vi "z_N[Lambda_tau,T,W,t_0]_Analytical.vi"(4 "Use z[0]":bool, 6 "t0":ext, 7 "Harmonic f":ext, 8 "N":i32, 9 "W":ext, 10 "T":ext, 11 "tau":ext) -> (3 "z_n,N,W(tau)":cxt)   [LabVIEW 2021, in "Phasor.lvlib"]
uses:
  Phasor.lvlib
  d7224bb0-7287-4d58-abbb-d1bd0f91def9.vi
  9cc972f5-8a98-42e2-8998-2ddda7d4f1f6.vi
  d7224bb0-7287-4d58-abbb-d1bd0f91def9.vi/8a80743f-1319-44c8-96b0-3ef8fc688731.vi
  d7224bb0-7287-4d58-abbb-d1bd0f91def9.vi/931f4f8f-d8c6-4056-833f-5c8fe97b24b9.vi
  9cc972f5-8a98-42e2-8998-2ddda7d4f1f6.vi/8a80743f-1319-44c8-96b0-3ef8fc688731.vi
  9cc972f5-8a98-42e2-8998-2ddda7d4f1f6.vi/931f4f8f-d8c6-4056-833f-5c8fe97b24b9.vi
  Math/ix/ix (EXT).vi
  Math/Math.lvlib
  22872093-43a4-40af-9bc9-9c64a134b50d.vi
  14c61276-7c1d-4dbf-adfa-5aadda4cd48c.vi
  51be3234-f280-4696-b9d2-a53dd0ed5f61.vi
  cc992cef-98b9-4ce6-98ee-904778ecd6ff.vi
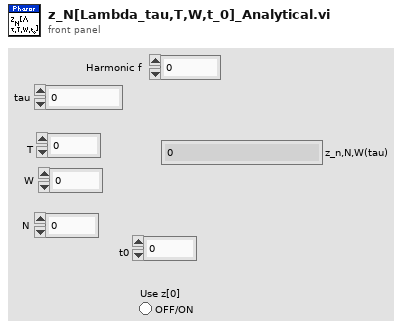
[diagram p1: front panel]
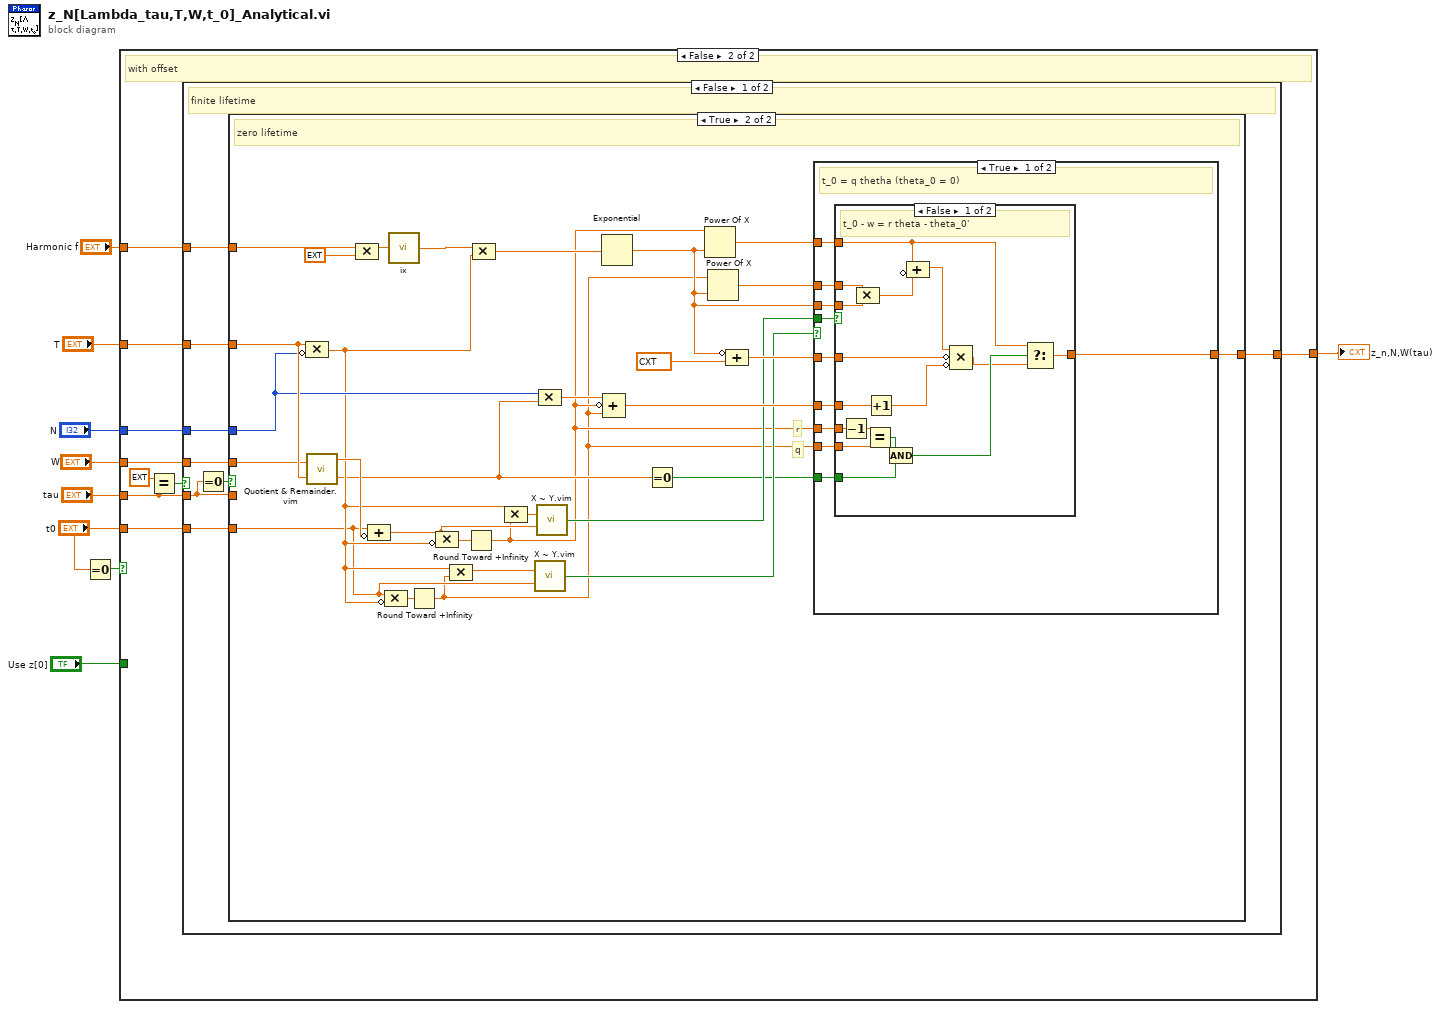
[diagram p0: block diagram]
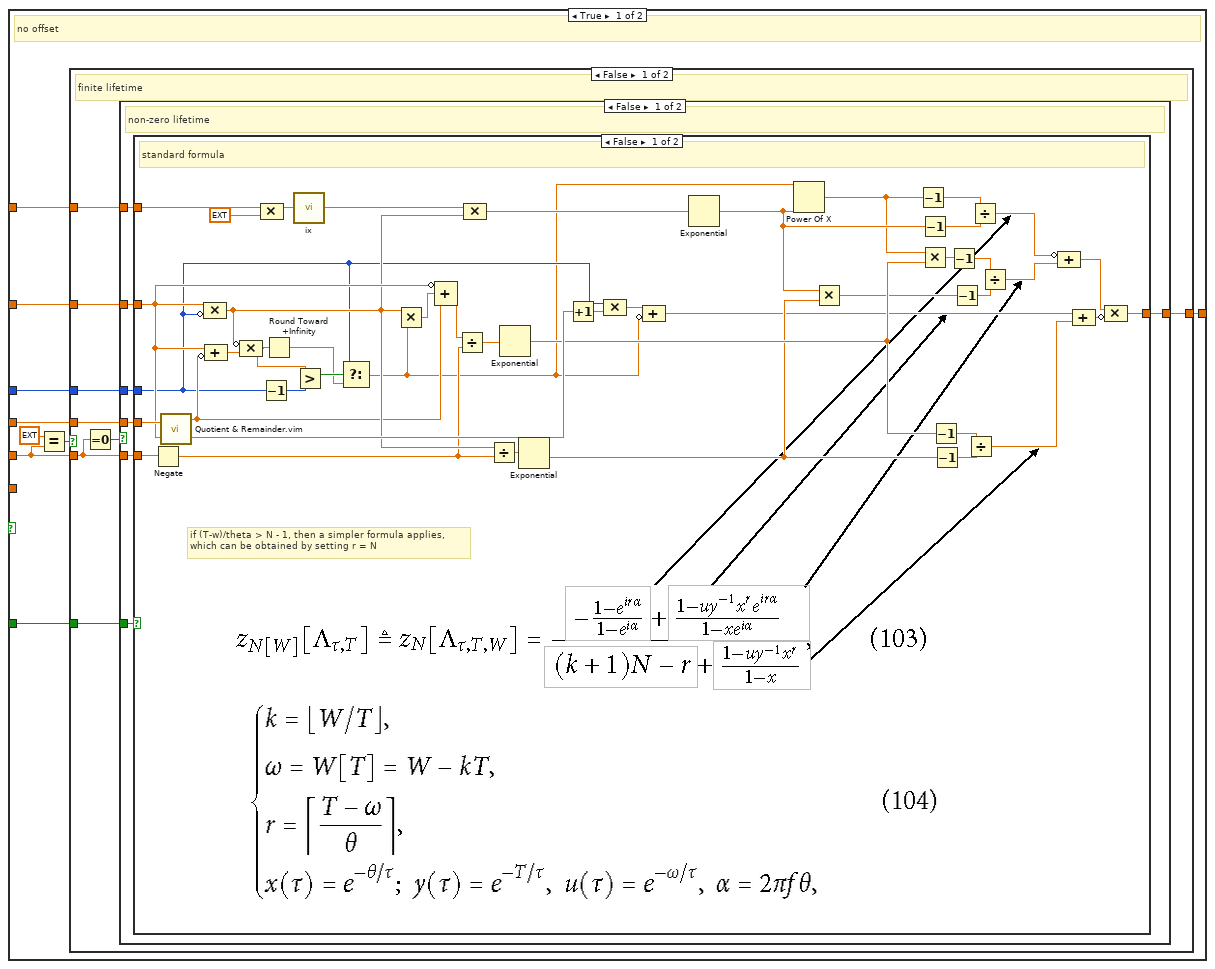
[diagram p2: hidden frame]
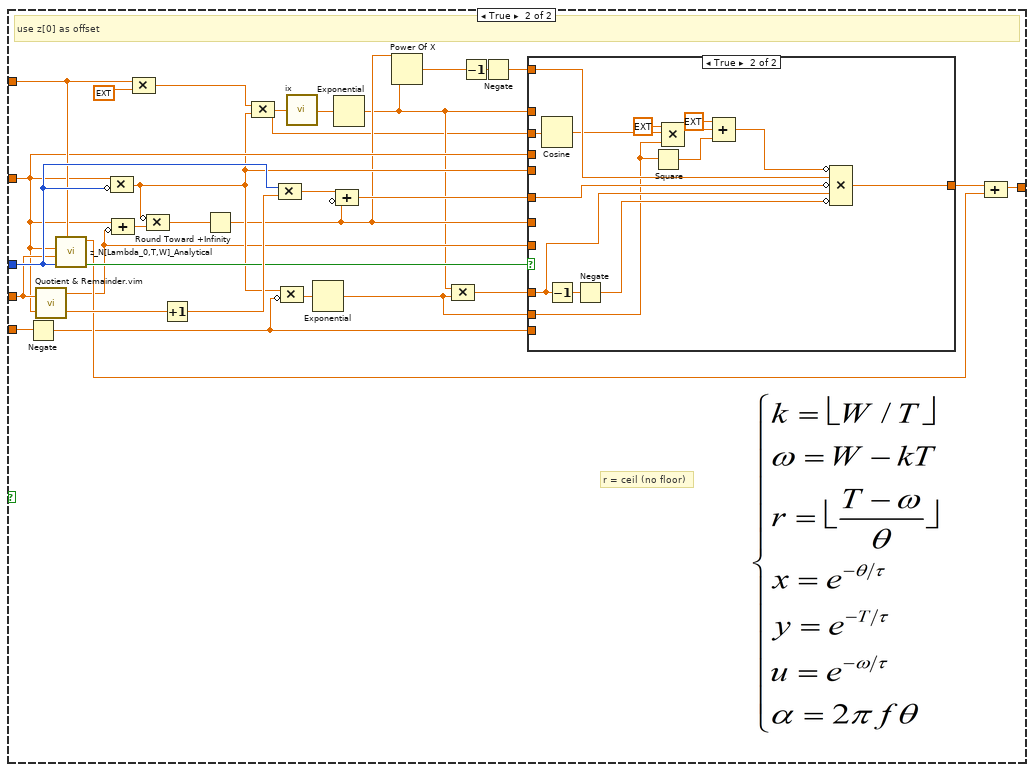
[diagram p3: hidden frame]
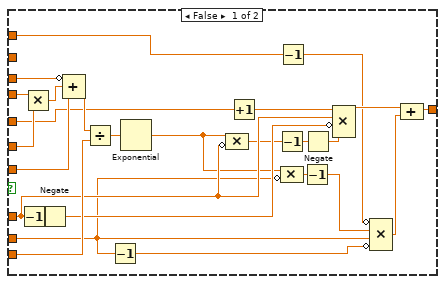
[diagram p4: hidden frame]
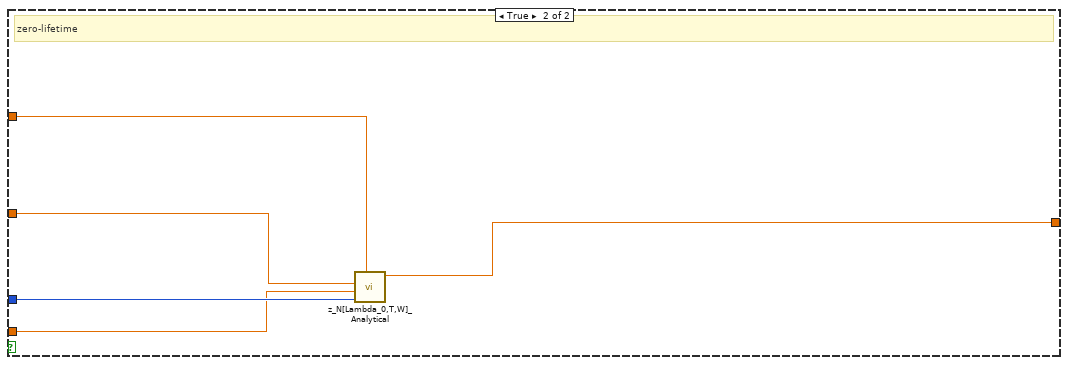
[diagram p5: hidden frame]
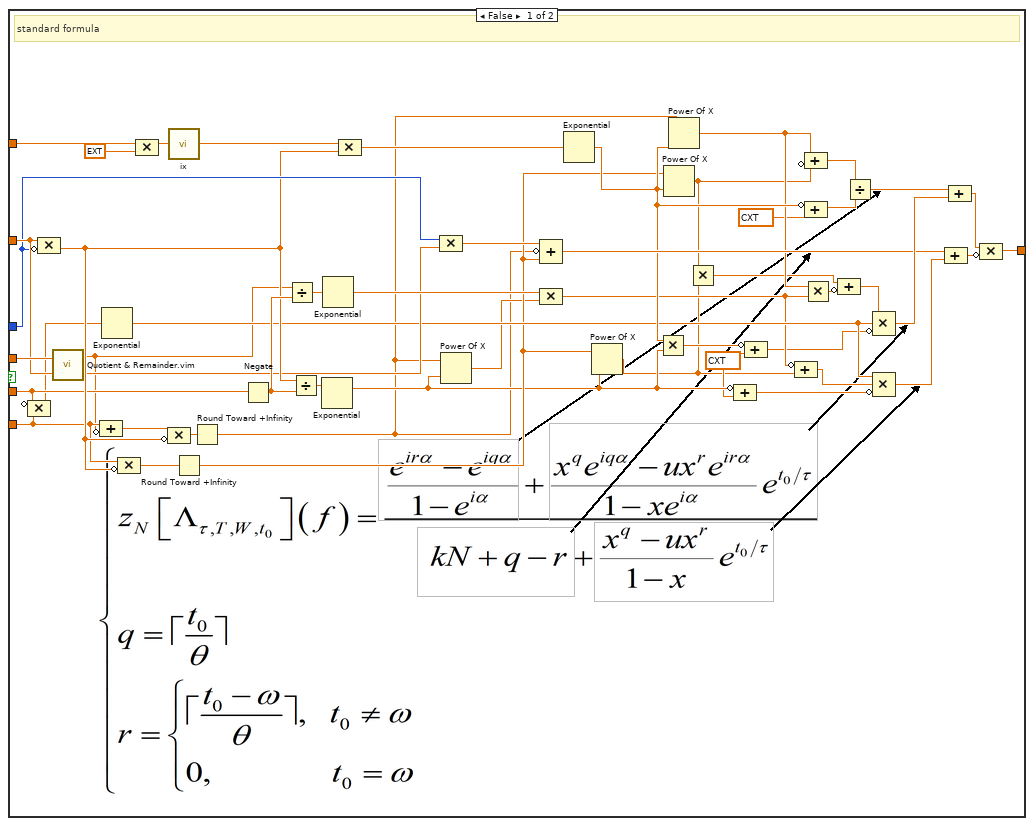
[diagram p7: hidden frame]
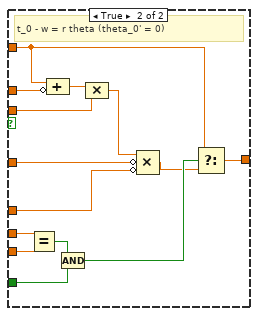
[diagram p8: hidden frame]
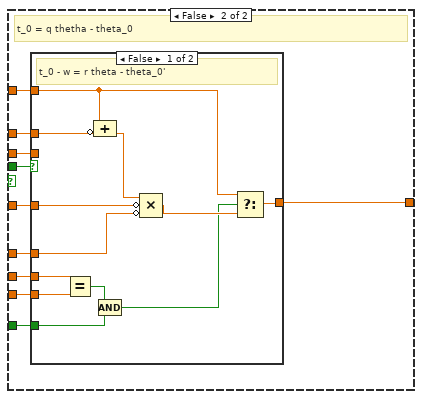
[diagram p9: hidden frame]
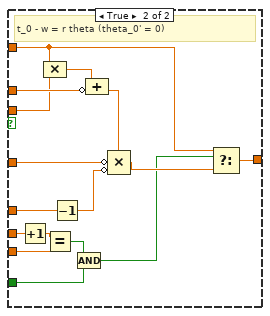
[diagram p10: hidden frame]
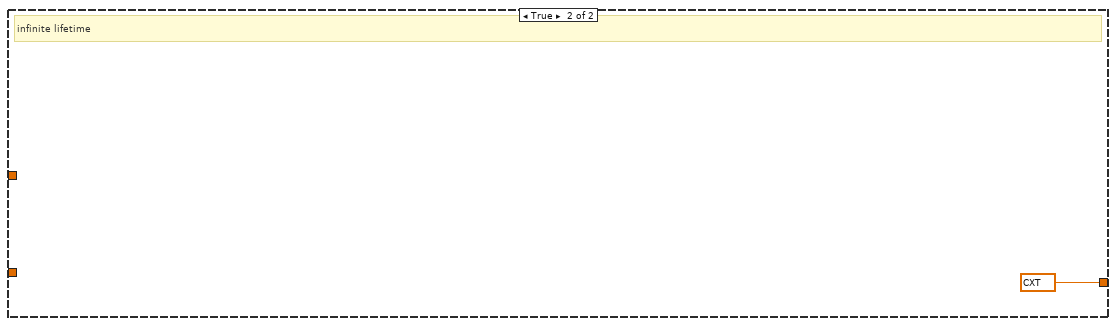
[diagram p11: hidden frame]
diagram:
  n1 = Equal To 0?(x="t0") -> (x = 0?=w2:bool)
  n2 = case shown="False" w2 {
    tunnel: "tau" -> [w13 w159]
    tunnel: "Harmonic f" -> [w18 w157]
    tunnel: [w17 w158] -> w7
    tunnel: "W" -> [w16 w156]
    tunnel: "T" -> [w14 w155]
    tunnel: "N" -> [w15 w154]
    tunnel: "t0" -> [_ w153]
    tunnel: "Use z[0]" -> [w10 _]
    frame True {
      # "no offset"
      n3 = Equal?(x=ext inf, y=w13) -> (x = y?=w11:bool)
      n4 = case shown="False" w11 {
        tunnel: w18 -> [w21 _]
        tunnel: [w26 _] -> w17
        tunnel: w16 -> [w25 _]
        tunnel: w15 -> [w24 _]
        tunnel: w14 -> [w23 _]
        tunnel: w13 -> [w22 _]
        tunnel: w10 -> [w19 _]
        frame False {
          # "finite lifetime"
          n5 = Equal To 0?(x=w22) -> (x = 0?=w20:bool)
          n6 = case shown="False" w20 {
            tunnel: [w33 w151] -> w26
            tunnel: w25 -> [w32 w148]
            tunnel: w24 -> [w31 w152]
            tunnel: w23 -> [w30 w149]
            tunnel: w22 -> [w29 _]
            tunnel: w21 -> [w28 w150]
            tunnel: w19 -> [w27 _]
            frame False {
              # "non-zero lifetime"
              n7 = case shown="False" w27 {
                tunnel: [w77 w93] -> w33
                tunnel: w32 -> [w76 w96]
                tunnel: w31 -> [w49 w98]
                tunnel: w30 -> [w60 w86]
                tunnel: w29 -> [w57 w101]
                tunnel: w28 -> [w46 w97]
                frame False {
                  # "if (T-w)/theta > N - 1, then a simpler formula applies,\nwhich can be obtained by setting r = N"
                  # "standard formula"
                  n8 = Negate(x=w57) -> (-x=w54:ext)
                  n9 = call "Quotient & Remainder.vim"("y"=w60, "x"=w76) -> ("E(x/y)"=w75:ext, "x - E(x/y)y"=w55:ext)
                  n10 = Compound Arithmetic op=MULTIPLY(w60, invert w49) -> (w58:ext)
                  n11 = Compound Arithmetic op=ADD(w60, invert w55) -> (w56:ext)
                  n12 = Compound Arithmetic op=MULTIPLY(invert w58, w56) -> (w47:ext)
                  n13 = Compound Arithmetic op=MULTIPLY(w46, ext 6.283185307179586477) -> (w45:ext)
                  n14 = Decrement(x=w49) -> (x-1=w52:i32)
                  n15 = Round Toward +Infinity(x=w47) -> (ceil(x): smallest int >= x=w50:ext)
                  n16 = call-poly "ix.vi"("x (1)"=w45) -> ("i.(x)"=w44:cxt)
                  n17 = Greater?(x=w47, y=w52) -> (0:w51:bool)
                  n18 = Select(t=w49, s=w51, f=w50) -> (s? t:f=w48:ext)
                  n19 = Multiply(x=w58, y=w48) -> (x*y=w43:ext)
                  n20 = Compound Arithmetic op=ADD(invert w60, w43, w55) -> (w42:ext)
                  n21 = Divide(x=w42, y=w54) -> (x/y=w41:ext)
                  n22 = Compound Arithmetic op=MULTIPLY(w44, w58) -> (w59:cxt)
                  n23 = Divide(x=w58, y=w54) -> (x/y=w40:ext)
                  n24 = Exponential(1:w41) -> (0:w72:ext)
                  n25 = Exponential(1:w40) -> (0:w69:ext)
                  n26 = Increment(x=w75) -> (x+1=w68:ext)
                  n27 = Compound Arithmetic op=MULTIPLY(w49, w68) -> (w67:ext)
                  n28 = Compound Arithmetic op=ADD(w67, invert w48) -> (w66:ext)
                  n29 = Exponential(1:w59) -> (0:w65:cxt)
                  n30 = Power Of X(1:w65, 2:w48) -> (0:w63:cxt)
                  n31 = Multiply(x=w65, y=w69) -> (x*y=w37:cxt)
                  n32 = Decrement(x=w63) -> (x-1=w53:cxt)
                  n33 = Decrement(x=w65) -> (x-1=w64:cxt)
                  n34 = Multiply(x=w63, y=w72) -> (x*y=w36:cxt)
                  n35 = Decrement(x=w72) -> (x-1=w35:ext)
                  n36 = Decrement(x=w69) -> (x-1=w34:ext)
                  n37 = Decrement(x=w36) -> (x-1=w39:cxt)
                  n38 = Decrement(x=w37) -> (x-1=w38:cxt)
                  n39 = Divide(x=w35, y=w34) -> (x/y=w71:ext)
                  n40 = Divide(x=w53, y=w64) -> (x/y=w62:cxt)
                  n41 = Divide(x=w39, y=w38) -> (x/y=w74:cxt)
                  n42 = Compound Arithmetic op=ADD(invert w62, w74) -> (w73:cxt)
                  n43 = Compound Arithmetic op=ADD(w66, w71) -> (w61:ext)
                  n44 = Compound Arithmetic op=MULTIPLY(w73, invert w61) -> (w77:cxt)
                }
                frame True {
                  # "r = ceil (no floor)"
                  # "use z[0] as offset"
                  n45 = Negate(x=w101) -> (-x=w82:ext)
                  n46 = call "Quotient & Remainder.vim"("y"=w86, "x"=w96) -> ("E(x/y)"=w107:ext, "x - E(x/y)y"=w83:ext)
                  n47 = call "z_N[Lambda_0,T,W]_Analytical.vi"("Harmonic f"=w97, "N"=w98, "W"=w96, "T"=w86) -> ("(T-w)/theta integer"=w95:bool, "z_n,N,W(0)"=w94:cxt)  [unwired: 6 in]
                  n48 = Compound Arithmetic op=MULTIPLY(w86, invert w98) -> (w85:ext)
                  n49 = Compound Arithmetic op=ADD(w86, invert w83) -> (w100:ext)
                  n50 = Compound Arithmetic op=MULTIPLY(w97, ext 6.283185307179586477) -> (w102:ext)
                  n51 = Compound Arithmetic op=MULTIPLY(invert w85, w100) -> (w99:ext)
                  n52 = Increment(x=w107) -> (x+1=w105:ext)
                  n53 = Round Toward +Infinity(x=w99) -> (ceil(x): smallest int >= x=w84:ext)
                  n54 = Compound Arithmetic op=MULTIPLY(w102, w85) -> (w79:ext)
                  n55 = Compound Arithmetic op=MULTIPLY(w98, w105) -> (w104:ext)
                  n56 = Compound Arithmetic op=MULTIPLY(w85, invert w82) -> (w89:ext)
                  n57 = call-poly "ix.vi"("x (1)"=w79) -> ("i.(x)"=w78:cxt)
                  n58 = Exponential(1:w89) -> (0:w81:ext)
                  n59 = Exponential(1:w78) -> (0:w80:cxt)
                  n60 = Compound Arithmetic op=ADD(w104, invert w84) -> (w91:ext)
                  n61 = Power Of X(1:w80, 2:w84) -> (0:w103:cxt)
                  n62 = Compound Arithmetic op=MULTIPLY(w80, w81) -> (w88:cxt)
                  n63 = Decrement(x=w103) -> (x-1=w92:cxt)
                  n64 = Negate(x=w92) -> (-x=w90:cxt)
                  n65 = case shown="True" w95 {
                    tunnel: w90 -> [_ w147]
                    tunnel: w91 -> [w125 w146]
                    tunnel: w88 -> [w121 w143]
                    tunnel: [w116 w142] -> w87
                    tunnel: w86 -> [w133 _]
                    tunnel: w85 -> [w132 _]
                    tunnel: w84 -> [w126 _]
                    tunnel: w83 -> [w131 _]
                    tunnel: w82 -> [w130 _]
                    tunnel: w81 -> [w112 w136]
                    tunnel: w80 -> [w113 _]
                    tunnel: w79 -> [_ w141]
                    frame False {
                      n66 = Decrement(x=w121) -> (x-1=w123:cxt)
                      n67 = Multiply(x=w132, y=w126) -> (x*y=w129:ext)
                      n68 = Negate(x=w123) -> (-x=w122:cxt)
                      n69 = Compound Arithmetic op=ADD(invert w133, w129, w131) -> (w128:ext)
                      n70 = Divide(x=w128, y=w130) -> (x/y=w127:ext)
                      n71 = Decrement(x=w112) -> (x-1=w111:ext)
                      n72 = Exponential(1:w127) -> (0:w115:ext)
                      n73 = Compound Arithmetic op=MULTIPLY(w115, invert w121) -> (w119:cxt)
                      n74 = Increment(x=w125) -> (x+1=w124:ext)
                      n75 = Decrement(x=w119) -> (x-1=w120:cxt)
                      n76 = Decrement(x=w113) -> (x-1=w108:cxt)
                      n77 = Compound Arithmetic op=MULTIPLY(w115, invert w112) -> (w114:ext)
                      n78 = Decrement(x=w114) -> (x-1=w109:ext)
                      n79 = Negate(x=w120) -> (-x=w118:cxt)
                      n80 = Compound Arithmetic op=MULTIPLY(w124, w121, invert w122, w118) -> (w117:cxt)
                      n81 = Compound Arithmetic op=MULTIPLY(invert w108, w109, w112, invert w111) -> (w110:cxt)
                      n82 = Compound Arithmetic op=ADD(w117, w110) -> (w116:cxt)
                    }
                    frame True {
                      n83 = Cosine(x=w141) -> (cos(x)=w140:ext)
                      n84 = Decrement(x=w143) -> (x-1=w145:cxt)
                      n85 = Negate(x=w145) -> (-x=w144:cxt)
                      n86 = Square(x=w136) -> (x^2=w135:ext)
                      n87 = Compound Arithmetic op=MULTIPLY(ext -2.0 ("value"), w140, w136) -> (w138:ext)
                      n88 = Compound Arithmetic op=ADD(ext 1.0 ("value"), w138, w135) -> (w134:ext)
                      n89 = Compound Arithmetic op=MULTIPLY(invert w134, w147, invert w146, w143, invert w144) -> (w142:cxt)
                    }
                  }
                  n90 = Compound Arithmetic op=ADD(w87, w94) -> (w93:cxt)
                }
              }
            }
            frame True {
              # "zero-lifetime"
              n91 = call "z_N[Lambda_0,T,W]_Analytical.vi"("Harmonic f"=w150, "N"=w152, "W"=w148, "T"=w149) -> ("z_n,N,W(0)"=w151:cxt)  [unwired: 6 in, 1 out]
            }
          }
        }
        frame True {
          # "infinite lifetime"
        }
      }
    }
    frame False {
      # "with offset"
      n92 = Equal?(x=ext inf, y=w159) -> (x = y?=w160:bool)
      n93 = case shown="False" w160 {
        tunnel: w159 -> [w165 _]
        tunnel: [w163 cxt 0.0+0.0i ("z_n,N,W(0)")] -> w158
        tunnel: w157 -> [w168 _]
        tunnel: w156 -> [w167 _]
        tunnel: w155 -> [w166 _]
        tunnel: w154 -> [w164 _]
        tunnel: w153 -> [w162 _]
        frame False {
          # "finite lifetime"
          n94 = Equal To 0?(x=w165) -> (x = 0?=w169:bool)
          n95 = case shown="True" w169 {
            tunnel: [w219 w221] -> w163
            tunnel: w167 -> [w218 w220]
            tunnel: w164 -> [w204 w245]
            tunnel: w166 -> [w207 w247]
            tunnel: w165 -> [w188 _]
            tunnel: w168 -> [w203 w244]
            tunnel: w162 -> [w187 w232]
            frame False {
              w176 = cxt 1.0+0.0i ("value")
              # "standard formula"
              n96 = Compound Arithmetic op=MULTIPLY(invert w188, w187) -> (w186:ext)
              n97 = Compound Arithmetic op=MULTIPLY(w207, invert w204) -> (w196:ext)
              n98 = call "Quotient & Remainder.vim"("y"=w207, "x"=w218) -> ("E(x/y)"=w189:ext, "x - E(x/y)y"=w182:ext)
              n99 = Compound Arithmetic op=ADD(w187, invert w182) -> (w194:ext)
              n100 = Exponential(1:w186) -> (0:w184:ext)
              n101 = Compound Arithmetic op=MULTIPLY(w187, invert w196) -> (w197:ext)
              n102 = Compound Arithmetic op=MULTIPLY(w203, ext 6.283185307179586477) -> (w202:ext)
              n103 = Compound Arithmetic op=MULTIPLY(w194, invert w196) -> (w195:ext)
              n104 = call-poly "ix.vi"("x (1)"=w202) -> ("i.(x)"=w201:cxt)
              n105 = Round Toward +Infinity(x=w197) -> (ceil(x): smallest int >= x=w183:ext)
              n106 = Round Toward +Infinity(x=w195) -> (ceil(x): smallest int >= x=w170:ext)
              n107 = Negate(x=w188) -> (-x=w205:ext)
              n108 = Divide(x=w182, y=w205) -> (x/y=w200:ext)
              n109 = Divide(x=w196, y=w205) -> (x/y=w199:ext)
              n110 = Exponential(1:w199) -> (0:w181:ext)
              n111 = Exponential(1:w200) -> (0:w215:ext)
              n112 = Compound Arithmetic op=MULTIPLY(w201, w196) -> (w206:cxt)
              n113 = Compound Arithmetic op=MULTIPLY(w204, w189) -> (w212:ext)
              n114 = Power Of X(1:w181, 2:w170) -> (0:w179:ext)
              n115 = Compound Arithmetic op=ADD(w212, invert w170, w183) -> (w211:ext)
              n116 = Compound Arithmetic op=MULTIPLY(w215, w179) -> (w180:ext)
              n117 = Exponential(1:w206) -> (0:w193:cxt)
              n118 = Power Of X(1:w181, 2:w183) -> (0:w174:ext)
              n119 = Multiply(x=w193, y=w181) -> (x*y=w178:cxt)
              n120 = Power Of X(1:w193, 2:w183) -> (0:w175:cxt)
              n121 = Power Of X(1:w193, 2:w170) -> (0:w192:cxt)
              n122 = Multiply(x=w175, y=w174) -> (x*y=w172:cxt)
              n123 = Compound Arithmetic op=unknown(invert w181, w176) -> (w198:cxt)
              n124 = Compound Arithmetic op=ADD(invert w178, w176) -> (w177:cxt)
              n125 = Compound Arithmetic op=ADD(invert w180, w174) -> (w185:ext)
              n126 = Multiply(x=w192, y=w180) -> (x*y=w173:cxt)
              n127 = Compound Arithmetic op=ADD(w192, invert w175) -> (w191:cxt)
              n128 = Compound Arithmetic op=ADD(invert w193, cxt 1.0+0.0i ("value")) -> (w210:cxt)
              n129 = Compound Arithmetic op=ADD(w172, invert w173) -> (w171:cxt)
              n130 = Divide(x=w191, y=w210) -> (x/y=w209:cxt)
              n131 = Compound Arithmetic op=MULTIPLY(w171, w184, invert w177) -> (w217:cxt)
              n132 = Compound Arithmetic op=MULTIPLY(w184, w185, invert w198) -> (w214:cxt)
              n133 = Compound Arithmetic op=ADD(w211, w214) -> (w208:cxt)
              n134 = Compound Arithmetic op=ADD(w209, w217) -> (w216:cxt)
              n135 = Compound Arithmetic op=MULTIPLY(w216, invert w208) -> (w219:cxt)
            }
            frame True {
              # "q"
              # "r"
              # "zero lifetime"
              n136 = Compound Arithmetic op=MULTIPLY(w247, invert w245) -> (w233:ext)
              n137 = call "Quotient & Remainder.vim"("y"=w247, "x"=w220) -> ("E(x/y)"=w225:ext, "x - E(x/y)y"=w238:ext)
              n138 = Compound Arithmetic op=MULTIPLY(w244, ext 6.283185307179586477) -> (w243:ext)
              n139 = Compound Arithmetic op=ADD(w232, invert w238) -> (w234:ext)
              n140 = Compound Arithmetic op=MULTIPLY(w232, invert w233) -> (w241:ext)
              n141 = call-poly "ix.vi"("x (1)"=w243) -> ("i.(x)"=w242:cxt)
              n142 = Round Toward +Infinity(x=w241) -> (ceil(x): smallest int >= x=w222:ext)
              n143 = Compound Arithmetic op=MULTIPLY(w234, invert w233) -> (w240:ext)
              n144 = Compound Arithmetic op=MULTIPLY(w233, w222) -> (w231:ext)
              n145 = Round Toward +Infinity(x=w240) -> (ceil(x): smallest int >= x=w223:ext)
              n146 = Compound Arithmetic op=MULTIPLY(w242, w233) -> (w246:cxt)
              n147 = Compound Arithmetic op=MULTIPLY(w233, w223) -> (w235:ext)
              n148 = call "X ~ Y.vim"("X"=w231, "Y"=w232) -> ("X ~= Y?"=w228:bool)  [unwired: 13 in]
              n149 = call "X ~ Y.vim"("X"=w235, "Y"=w234) -> ("X ~= Y?"=w227:bool)  [unwired: 13 in]
              n150 = Compound Arithmetic op=MULTIPLY(w245, w225) -> (w248:ext)
              n151 = Exponential(1:w246) -> (0:w226:cxt)
              n152 = Compound Arithmetic op=ADD(w248, invert w223, w222) -> (w236:ext)
              n153 = Equal To 0?(x=w225) -> (x = 0?=w224:bool)
              n154 = Power Of X(1:w226, 2:w223) -> (0:w239:cxt)
              n155 = Power Of X(1:w226, 2:w222) -> (0:w237:cxt)
              n156 = Compound Arithmetic op=ADD(invert w226, cxt 1.0+0.0i ("value")) -> (w229:cxt)
              n157 = case shown="True" w228 {
                tunnel: w239 -> [w259 w299]
                tunnel: w237 -> [w258 w298]
                tunnel: w227 -> [w257 w297]
                tunnel: w226 -> [w256 w296]
                tunnel: w236 -> [w254 w291]
                tunnel: w229 -> [w255 w292]
                tunnel: w224 -> [w251 w295]
                tunnel: w223 -> [w253 w294]
                tunnel: w222 -> [w252 w293]
                tunnel: [w250 w290] -> w221
                frame True {
                  # "t_0 = q thetha (theta_0 = 0)"
                  n158 = case shown="False" w257 {
                    tunnel: w259 -> [w261 w276]
                    tunnel: w258 -> [w275 w289]
                    tunnel: w256 -> [w274 w287]
                    tunnel: w255 -> [w271 w281]
                    tunnel: w254 -> [w270 w280]
                    tunnel: w253 -> [w266 w286]
                    tunnel: w252 -> [w265 w285]
                    tunnel: w251 -> [w264 w283]
                    tunnel: [w268 w278] -> w250
                    frame False {
                      # "t_0 - w = r theta - theta_0'"
                      n159 = Decrement(x=w266) -> (x-1=w260:ext)
                      n160 = Compound Arithmetic op=MULTIPLY(w275, w274) -> (w273:cxt)
                      n161 = Equal?(x=w260, y=w265) -> (x = y?=w267:bool)
                      n162 = Increment(x=w270) -> (x+1=w269:ext)
                      n163 = Compound Arithmetic op=AND(w267, w264) -> (w263:bool)
                      n164 = Compound Arithmetic op=ADD(w261, invert w273) -> (w272:cxt)
                      n165 = Compound Arithmetic op=MULTIPLY(w272, invert w271, invert w269) -> (w262:cxt)
                      n166 = Select(t=w261, s=w263, f=w262) -> (s? t:f=w268:cxt)
                    }
                    frame True {
                      # "t_0 - w = r theta (theta_0' = 0)"
                      n167 = Equal?(x=w286, y=w285) -> (x = y?=w284:bool)
                      n168 = Compound Arithmetic op=ADD(w276, invert w289) -> (w288:cxt)
                      n169 = Compound Arithmetic op=AND(w284, w283) -> (w279:bool)
                      n170 = Compound Arithmetic op=MULTIPLY(w288, w287) -> (w282:cxt)
                      n171 = Compound Arithmetic op=MULTIPLY(w282, invert w281, invert w280) -> (w277:cxt)
                      n172 = Select(t=w276, s=w279, f=w277) -> (s? t:f=w278:cxt)
                    }
                  }
                }
                frame False {
                  # "t_0 = q thetha - theta_0"
                  n173 = case shown="False" w297 {
                    tunnel: w299 -> [w306 w313]
                    tunnel: w298 -> [w311 w327]
                    tunnel: w296 -> [_ w326]
                    tunnel: w295 -> [w303 w315]
                    tunnel: w294 -> [w301 w318]
                    tunnel: w293 -> [w300 w317]
                    tunnel: w292 -> [w309 w323]
                    tunnel: w291 -> [w308 w322]
                    tunnel: [w307 w312] -> w290
                    frame False {
                      # "t_0 - w = r theta - theta_0'"
                      n174 = Equal?(x=w301, y=w300) -> (x = y?=w304:bool)
                      n175 = Compound Arithmetic op=ADD(w306, invert w311) -> (w310:cxt)
                      n176 = Compound Arithmetic op=AND(w304, w303) -> (w302:bool)
                      n177 = Compound Arithmetic op=MULTIPLY(w310, invert w309, invert w308) -> (w305:cxt)
                      n178 = Select(t=w306, s=w302, f=w305) -> (s? t:f=w307:cxt)
                    }
                    frame True {
                      # "t_0 - w = r theta (theta_0' = 0)"
                      n179 = Increment(x=w318) -> (x+1=w316:ext)
                      n180 = Compound Arithmetic op=MULTIPLY(w313, w326) -> (w325:cxt)
                      n181 = Equal?(x=w316, y=w317) -> (x = y?=w319:bool)
                      n182 = Decrement(x=w322) -> (x-1=w321:ext)
                      n183 = Compound Arithmetic op=AND(w319, w315) -> (w314:bool)
                      n184 = Compound Arithmetic op=ADD(w325, invert w327) -> (w324:cxt)
                      n185 = Compound Arithmetic op=MULTIPLY(w324, invert w323, invert w321) -> (w320:cxt)
                      n186 = Select(t=w313, s=w314, f=w320) -> (s? t:f=w312:cxt)
                    }
                  }
                }
              }
            }
          }
        }
        frame True {
          # "infinite lifetime"
        }
      }
    }
  }
  "z_n,N,W(tau)" <- w7
